vi "tm3samp_09_lightsheet.vi"() -> ()   [LabVIEW 2011]
panel:
  in  "Input Trigger Polarity":u32(ring)=1 items=["NEGATIVE"=1, "POSITIVE"=2]
  in  "Input Trigger Mode":u32(ring)=1 items=["INTERNAL"=1, "EXTERNAL EDGE"=2, "EXTERNAL LEVEL"=4, "SOFTWARE"=32, "FAST REPETITION"=64, "TDI"=128, "START"=512, "SYNC READOUT"=1024]
  in  "Internal Line Speed":dbl=0.5
  in  "Output Trigger Period":dbl=1e-05
  in  "Output Trigger Polarity":u32(ring)=1 items=["NEGATIVE"=1, "POSITIVE"=2]
  in  "Output Trigger Mode":u32(ring)=3 items=["LOW"=1, "GLOBAL EXPOSURE"=2, "PROGRAMMABLE"=3, "TRIGGER READY"=4, "HIGH"=5]
  in  "Readout Direction":u32(ring)=1 items=["FORWARD"=1, "BACKWARD"=2]
  in  "Pre Hsync Count":u32
  out "Image":u16[][](graph)
  out "Frames Per Second":dbl
  in  "Quit":bool
  out "Error Out":errorcluster {"code" format="%.0x"}
  # "This is just a simple example\nof how to setup a camera for\na Lightsheet application with\na Flash4.0 V2"
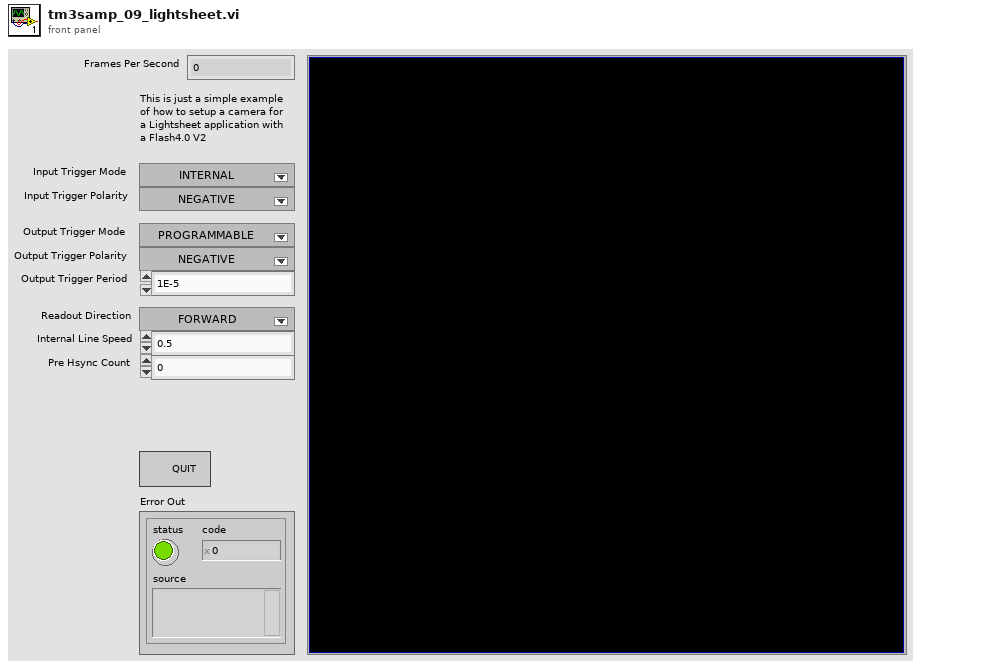
[diagram p1: front panel]
types:
  T1 = cluster{"Input Trigger Mode":u32, "Input Trigger Polarity":u32, "Times":u32, "Delay":dbl}
  T2 = cluster{"Output Trigger Mode":u32, "Output Trigger Polarity":u32, "Output Trigger Period":dbl, "Delay":dbl}
  T3 = cluster{"height":u32, "width":u32, "datatype":u32}
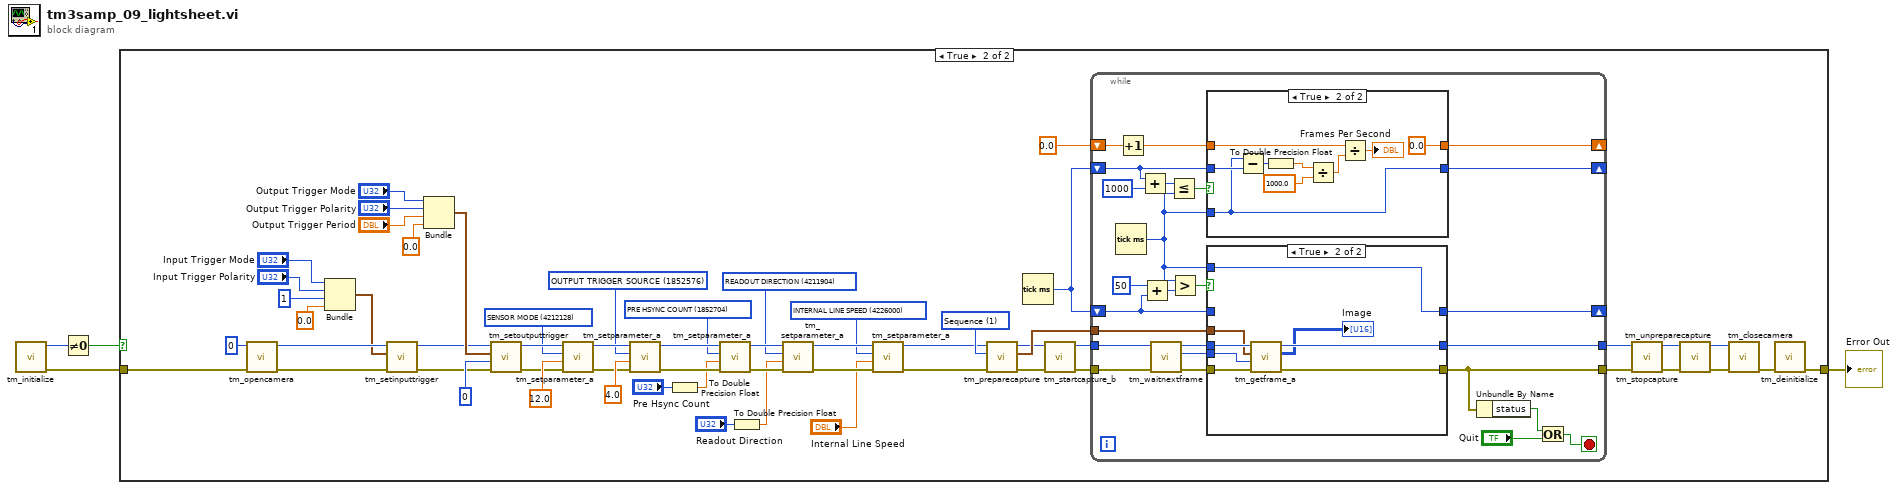
[diagram p0: block diagram]
diagram:
  n1 = call <userlib>:"tm_initialize.vi"() -> ("error out"=w1:errorcluster, "Number Of Cameras"=w2:u32)  [unwired: 8 in, 2 out]
  n2 = Not Equal To 0?(x=w2) -> (x != 0?=w4:bool)
  n3 = case shown="True" w4 {
    tunnel: w1 -> [w5 w62]
    tunnel: [w5 w59] -> w3
    frame False {
    }
    frame True {
      w11 = u32 4226000 items=["SENSOR MODE"=4212128, "CCD MODE"=4212384, "READOUT MODE"=4211872, "ACTIVE VIEW INDEX"=4343136, "BITS PER CHANNEL"=4342976, "IMAGE PIXEL TYPE"=4343296, "BINNING"=4215968, "EXPOSURE TIME"=2049184, "CONTRAST GAIN"=3163312, "CONTRAST OFFSET"=3163328, "LIGHT MODE"=2114720, "SENSITIVITY"=2114992, "PHOTON IMAGING MODE"=2115200, "HIGH DYNAMIC RANGE MODE"=3163360, "WHITE BALANCE"=3163568, "TEMPERATURE"=2115232, "TEMPERATURE TARGET"=2115264, "SENSOR COOLER FAN"=2115296, "LINEBUNDLE HEIGHT"=4212192, "MECHANICAL SHUTTER"=2115488, "BACK FOCUS POSITION"=8422304, "TRIGGER CONNECTOR"=1066432, "TRIGGER SOURCE"=1066144, "OUTPUT TRIGGER SOURCE"=1852576, "TRIGGER GLOBAL EXPOSURE"=2049680, "FIRST TRIGGER BEHAVIOR"=2049696, "CHANNEL SYNC"=1852352, "READOUT DIRECTION"=4211904, "PRE HSYNC COUNT"=1852704, "INTERNAL LINE SPEED"=4226000, "INTERNAL LINE INTERVAL"=4226016] ("Parameter")
      w17 = u32 4212128 items=["SENSOR MODE"=4212128, "CCD MODE"=4212384, "READOUT MODE"=4211872, "ACTIVE VIEW INDEX"=4343136, "BITS PER CHANNEL"=4342976, "IMAGE PIXEL TYPE"=4343296, "BINNING"=4215968, "EXPOSURE TIME"=2049184, "CONTRAST GAIN"=3163312, "CONTRAST OFFSET"=3163328, "LIGHT MODE"=2114720, "SENSITIVITY"=2114992, "PHOTON IMAGING MODE"=2115200, "HIGH DYNAMIC RANGE MODE"=3163360, "WHITE BALANCE"=3163568, "TEMPERATURE"=2115232, "TEMPERATURE TARGET"=2115264, "SENSOR COOLER FAN"=2115296, "LINEBUNDLE HEIGHT"=4212192, "MECHANICAL SHUTTER"=2115488, "BACK FOCUS POSITION"=8422304, "TRIGGER CONNECTOR"=1066432, "TRIGGER SOURCE"=1066144, "OUTPUT TRIGGER SOURCE"=1852576, "TRIGGER GLOBAL EXPOSURE"=2049680, "FIRST TRIGGER BEHAVIOR"=2049696, "CHANNEL SYNC"=1852352, "READOUT DIRECTION"=4211904, "PRE HSYNC COUNT"=1852704, "INTERNAL LINE SPEED"=4191408, "INTERNAL LINE INTERVAL"=4191424] ("Parameter")
      w18 = u32 1852576 items=["SENSOR MODE"=4212128, "CCD MODE"=4212384, "READOUT MODE"=4211872, "ACTIVE VIEW INDEX"=4343136, "BITS PER CHANNEL"=4342976, "IMAGE PIXEL TYPE"=4343296, "BINNING"=4215968, "EXPOSURE TIME"=2049184, "CONTRAST GAIN"=3163312, "CONTRAST OFFSET"=3163328, "LIGHT MODE"=2114720, "SENSITIVITY"=2114992, "PHOTON IMAGING MODE"=2115200, "HIGH DYNAMIC RANGE MODE"=3163360, "WHITE BALANCE"=3163568, "TEMPERATURE"=2115232, "TEMPERATURE TARGET"=2115264, "SENSOR COOLER FAN"=2115296, "LINEBUNDLE HEIGHT"=4212192, "MECHANICAL SHUTTER"=2115488, "BACK FOCUS POSITION"=8422304, "TRIGGER CONNECTOR"=1066432, "TRIGGER SOURCE"=1066144, "OUTPUT TRIGGER SOURCE"=1852576, "TRIGGER GLOBAL EXPOSURE"=2049680, "FIRST TRIGGER BEHAVIOR"=2049696, "CHANNEL SYNC"=1852352, "READOUT DIRECTION"=4211904, "PRE HSYNC COUNT"=1852704, "INTERNAL LINE SPEED"=4191408, "INTERNAL LINE INTERVAL"=4191424] ("Parameter")
      w19 = u32 1852704 items=["SENSOR MODE"=4212128, "CCD MODE"=4212384, "READOUT MODE"=4211872, "ACTIVE VIEW INDEX"=4343136, "BITS PER CHANNEL"=4342976, "IMAGE PIXEL TYPE"=4343296, "BINNING"=4215968, "EXPOSURE TIME"=2049184, "CONTRAST GAIN"=3163312, "CONTRAST OFFSET"=3163328, "LIGHT MODE"=2114720, "SENSITIVITY"=2114992, "PHOTON IMAGING MODE"=2115200, "HIGH DYNAMIC RANGE MODE"=3163360, "WHITE BALANCE"=3163568, "TEMPERATURE"=2115232, "TEMPERATURE TARGET"=2115264, "SENSOR COOLER FAN"=2115296, "LINEBUNDLE HEIGHT"=4212192, "MECHANICAL SHUTTER"=2115488, "BACK FOCUS POSITION"=8422304, "TRIGGER CONNECTOR"=1066432, "TRIGGER SOURCE"=1066144, "OUTPUT TRIGGER SOURCE"=1852576, "TRIGGER GLOBAL EXPOSURE"=2049680, "FIRST TRIGGER BEHAVIOR"=2049696, "CHANNEL SYNC"=1852352, "READOUT DIRECTION"=4211904, "PRE HSYNC COUNT"=1852704, "INTERNAL LINE SPEED"=4191408, "INTERNAL LINE INTERVAL"=4191424] ("Parameter")
      w20 = u32 4211904 items=["SENSOR MODE"=4212128, "CCD MODE"=4212384, "READOUT MODE"=4211872, "ACTIVE VIEW INDEX"=4343136, "BITS PER CHANNEL"=4342976, "IMAGE PIXEL TYPE"=4343296, "BINNING"=4215968, "EXPOSURE TIME"=2049184, "CONTRAST GAIN"=3163312, "CONTRAST OFFSET"=3163328, "LIGHT MODE"=2114720, "SENSITIVITY"=2114992, "PHOTON IMAGING MODE"=2115200, "HIGH DYNAMIC RANGE MODE"=3163360, "WHITE BALANCE"=3163568, "TEMPERATURE"=2115232, "TEMPERATURE TARGET"=2115264, "SENSOR COOLER FAN"=2115296, "LINEBUNDLE HEIGHT"=4212192, "MECHANICAL SHUTTER"=2115488, "BACK FOCUS POSITION"=8422304, "TRIGGER CONNECTOR"=1066432, "TRIGGER SOURCE"=1066144, "OUTPUT TRIGGER SOURCE"=1852576, "TRIGGER GLOBAL EXPOSURE"=2049680, "FIRST TRIGGER BEHAVIOR"=2049696, "CHANNEL SYNC"=1852352, "READOUT DIRECTION"=4211904, "PRE HSYNC COUNT"=1852704, "INTERNAL LINE SPEED"=4191408, "INTERNAL LINE INTERVAL"=4191424] ("Parameter")
      w50 = 1 items=["Snap", "Sequence"] ("Capture mode")
      n4 = call <userlib>:"tm_opencamera.vi"("error in (no error)"=w62, "Camera Index"=u32 0) -> ("error out"=w25:errorcluster, "Handle out"=w26:u32)  [unwired: 7 in, 1 out]
      n5 = Bundle("Input Trigger Mode"="Input Trigger Mode", "Input Trigger Polarity"="Input Trigger Polarity", "Times"=u32 1, "Delay"=0.0) -> (w10:T1)  [unwired: 1 in]
      n6 = call <userlib>:"tm_setinputtrigger.vi"("error in (no error)"=w25, "Parameters"=w10, "Handle in"=w26) -> ("error out"=w28:errorcluster, "Handle out"=w27:u32)  [unwired: 7 in]
      n7 = Bundle("Output Trigger Mode"="Output Trigger Mode", "Output Trigger Polarity"="Output Trigger Polarity", "Output Trigger Period"="Output Trigger Period", "Delay"=0.0) -> (w33:T2)  [unwired: 1 in]
      n8 = call <userlib>:"tm_setoutputtrigger.vi"("error in (no error)"=w28, "Index"=0, "Parameters"=w33, "Handle in"=w27) -> ("error out"=w23:errorcluster, "Handle out"=w24:u32)  [unwired: 6 in]
      n9 = call <userlib>:"tm_setparameter_a.vi"("error in (no error)"=w23, "Value in"=12.0, "Parameter"=w17, "Handle in"=w24) -> ("error out"=w21:errorcluster, "Handle out"=w22:u32)  [unwired: 6 in]
      n10 = call <userlib>:"tm_setparameter_a.vi"("error in (no error)"=w21, "Value in"=4.0, "Parameter"=w18, "Handle in"=w22) -> ("error out"=w41:errorcluster, "Handle out"=w42:u32)  [unwired: 6 in]
      n11 = To Double Precision Float(number="Pre Hsync Count") -> (double precision float=w40:dbl)
      n12 = call <userlib>:"tm_setparameter_a.vi"("error in (no error)"=w41, "Value in"=w40, "Parameter"=w19, "Handle in"=w42) -> ("error out"=w38:errorcluster, "Handle out"=w37:u32)  [unwired: 6 in]
      n13 = To Double Precision Float(number="Readout Direction") -> (double precision float=w36:dbl)
      n14 = call <userlib>:"tm_setparameter_a.vi"("error in (no error)"=w38, "Value in"=w36, "Parameter"=w20, "Handle in"=w37) -> ("error out"=w15:errorcluster, "Handle out"=w16:u32)  [unwired: 6 in]
      n15 = call <userlib>:"tm_setparameter_a.vi"("error in (no error)"=w15, "Value in"="Internal Line Speed", "Parameter"=w11, "Handle in"=w16) -> ("error out"=w13:errorcluster, "Handle out"=w12:u32)  [unwired: 6 in]
      n16 = call <userlib>:"tm_preparecapture.vi"("error in (no error)"=w13, "Capture mode"=w50, "Handle in"=w12) -> ("error out"=w47:errorcluster, "Buffer Info"=w49:T3, "Handle out"=w48:u32)  [unwired: 5 in, 1 out]
      n17 = Tick Count (ms)() -> (millisecond timer value=w45:u32)
      n18 = call <userlib>:"tm_startcapture_b.vi"("error in (no error)"=w47, "Handle in"=w48) -> ("error out"=w51:errorcluster, "Handle out"=w52:u32)  [unwired: 8 in]
      n19 = while {
        tunnel: [w66] -> w55
        tunnel: [w67] -> w56
        tunnel: w49 -> [w64]
        tunnel: w52 -> [w84]
        tunnel: w51 -> [w85]
        shift-right: [w82] -> _
        shift-left: w45 -> [w79]
        shift-right: [w83] -> _
        shift-left: 0.0 -> [w76]
        shift-right: [w65] -> _
        shift-left: w45 -> [w68]
        stop <- w63 stop-if-true
        n20 = Tick Count (ms)() -> (millisecond timer value=w69:u32)
        n21 = Increment(x=w76) -> (x+1=w77:dbl)
        n22 = Add(x=w79, y=u32 1000) -> (x+y=w81:u32)
        n23 = Add(x=u32 50, y=w68) -> (x+y=w71:u32)
        n24 = call <userlib>:"tm_waitnextframe.vi"("error in (no error)"=w85, "Handle in"=w84) -> ("error out"=w74:errorcluster, "Frame Index"=w73:i32, "Handle out"=w75:u32)  [unwired: 6 in, 1 out]
        n25 = Less Or Equal?(x=w81, y=w69) -> (x <= y?=w78:bool)
        n26 = Greater?(x=w69, y=w71) -> (0:w70:bool)
        n27 = case shown="True" w78 {
          tunnel: w79 -> [w100 w103]
          tunnel: [w100 w101] -> w82
          tunnel: w77 -> [w99 w107]
          tunnel: w69 -> [_ w101]
          tunnel: [w99 0.0] -> w83
          frame False {
          }
          frame True {
            n28 = Subtract(x=w101, y=w103) -> (x-y=w102:u32)
            n29 = To Double Precision Float(number=w102) -> (double precision float=w109:dbl)
            n30 = Divide(x=w109, y=1000.0) -> (x/y=w106:dbl)
            n31 = Divide(x=w107, y=w106) -> (x/y=→"Frames Per Second":dbl)
          }
        }
        n32 = case shown="True" w70 {
          tunnel: w75 -> [w90 w98]
          tunnel: w74 -> [w89 w97]
          tunnel: w73 -> [_ w96]
          tunnel: w68 -> [w88 _]
          tunnel: w69 -> [_ w95]
          tunnel: [w90 w92] -> w66
          tunnel: [w89 w93] -> w67
          tunnel: [w88 w95] -> w65
          tunnel: w64 -> [_ w94]
          frame False {
          }
          frame True {
            n33 = call <userlib>:"tm_getframe_a.vi"("error in (no error)"=w97, "Frame Index"=w96, "Buffer Info"=w94, "Handle in"=w98) -> ("error out"=w93:errorcluster, "Data 16"=→"Image":u16[][], "Handle out"=w92:u32)  [unwired: 3 in, 2 out]
          }
        }
        n34 = Unbundle By Name(w67) -> ("status"=w87:bool)
        n35 = Or(x=w87, y="Quit") -> (x .or. y?=w63:bool)
      }
      n36 = call <userlib>:"tm_stopcapture.vi"("error in (no error)"=w56, "Handle in"=w55) -> ("error out"=w53:errorcluster, "Handle out"=w54:u32)  [unwired: 8 in]
      n37 = call <userlib>:"tm_unpreparecapture.vi"("error in (no error)"=w53, "Handle in"=w54) -> ("error out"=w58:errorcluster, "Handle out"=w57:u32)  [unwired: 8 in]
      n38 = call <userlib>:"tm_closecamera.vi"("error in (no error)"=w58, "Handle in"=w57) -> ("error out"=w60:errorcluster)  [unwired: 9 in]
      n39 = call <userlib>:"tm_deinitialize.vi"("error in (no error)"=w60) -> ("error out"=w59:errorcluster)  [unwired: 10 in]
    }
  }
  "Error Out" <- w3
